vi "LAB4-2.vi"() -> ()   [LabVIEW 2011]
uses:
  <userlib>/KNR LabVIEW Toolkit/General/KNR Open (Direct Mode).vi
  <userlib>/KNR LabVIEW Toolkit/AI Control/AI Library.lvlib
panel:
  out "Voltages":dbl[](array[numeric])
  out "ADC Code":i16[](array[numeric])
  out "Voltage":dbl
  out "Distance (cm)":dbl
  in  "8-15 Single ended":bool=TRUE
  in  "0-7 Single ended":bool=TRUE
  out "error out":errorcluster
  in  "stop":bool
  # "Takes AI0 and converts voltage to distance.\n\n將超音波感測器接上AI0，選擇Sharp型號，\n並轉換為距離。"
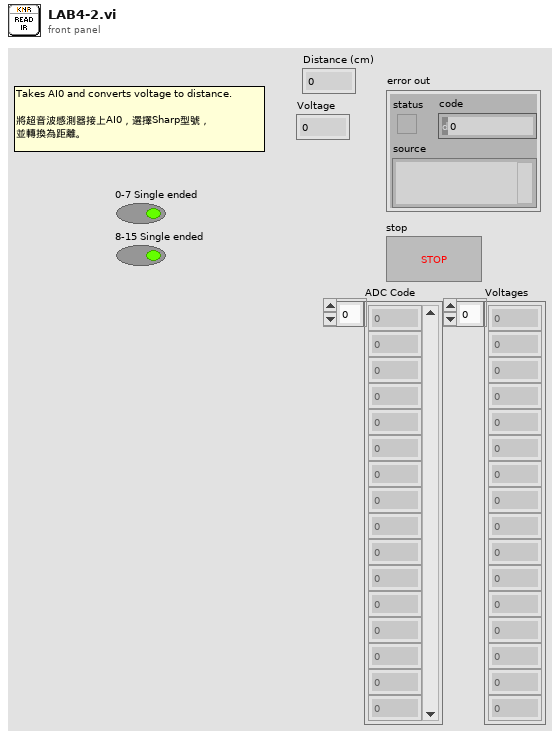
[diagram p1: front panel]
types:
  T1 = typedef "KNR Reference.ctl" = cluster{"FPGA Session":refnum<class "FPGA Interface Base.lvclass">, "Port Types":T2[]}
  T2 = typedef "Port Type (API).ctl" = enum8{"Unassigned", "DIO", "DC Motor", "RC Motor", "Ultrasonic", "Analog Input"}
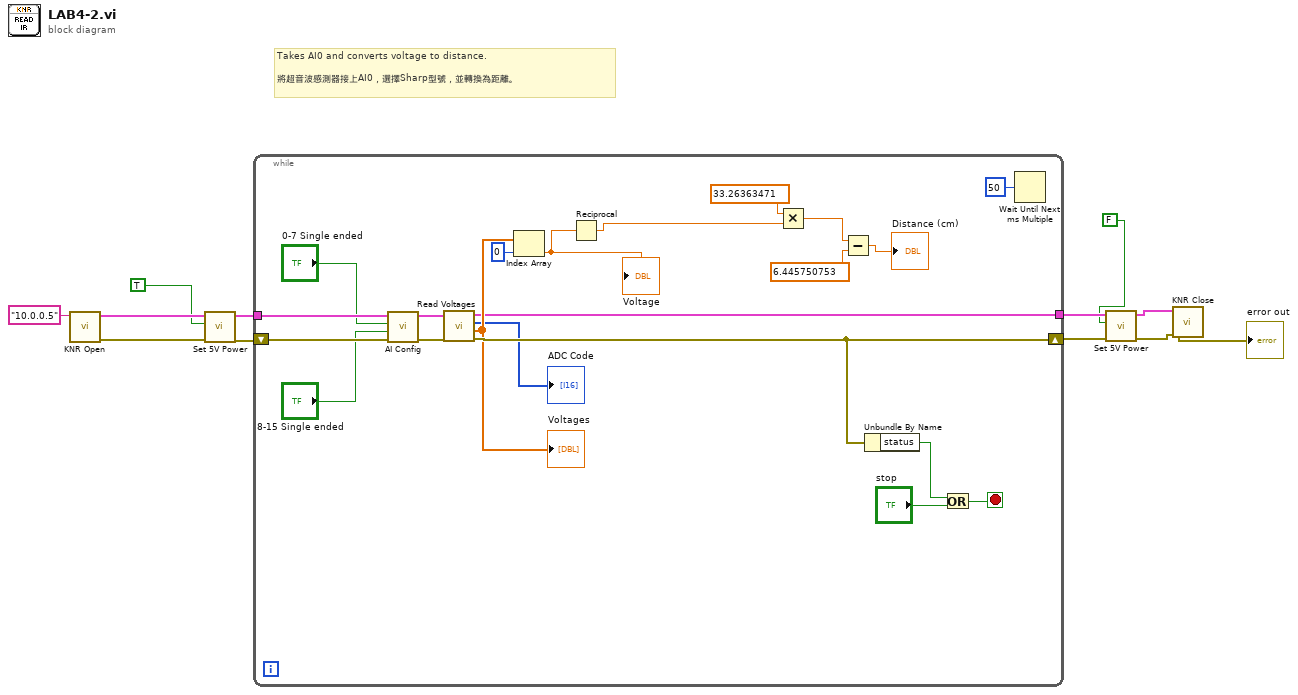
[diagram p0: block diagram]
diagram:
  # "Takes AI0 and converts voltage to distance.\n\n將超音波感測器接上AI0，選擇Sharp型號，並轉換為距離。"
  n1 = call-poly <userlib>:"KNR Open.vi"("IP Address (Default: 10.0.0.5)"="10.0.0.5") -> ("error out"=w11:errorcluster, "KNR Out"=w12:T1)  [unwired: 9 in]
  n2 = call <userlib>:"Set 5V Power.vi"("error in (no error)"=w11, "5V Power"=TRUE, "KNR In"=w12) -> ("error out"=w8:errorcluster, "KNR Out"=w9:T1)  [unwired: 7 in]
  n3 = while {
    tunnel: w9 -> [w29]
    shift-right: [w25] -> w2
    shift-left: w8 -> [w28]
    tunnel: [w14] -> w5
    stop <- w31 stop-if-true
    n4 = call <userlib>:"AI Config.vi"("error in (no error)"=w28, "8-15 Single ended"="8-15 Single ended", "0-7 Single ended"="0-7 Single ended", "KNR In"=w29) -> ("error out"=w26:errorcluster, "KNR Out"=w27:T1)  [unwired: 6 in]
    n5 = call <userlib>:"Read Voltages.vi"("error in (no error)"=w26, "KNR In"=w27) -> ("error out"=w25:errorcluster, "Voltages"=w22:dbl[], "ADC Code"=→"ADC Code":i16[], "KNR Out"=w14:T1)  [unwired: 6 in]
    "Voltages" <- w22
    n6 = Index Array(array=w22, index=0) -> (element=w20:dbl)
    "Voltage" <- w20
    n7 = Reciprocal(x=w20) -> (1/x=w15:dbl)
    n8 = Multiply(x=33.26363471, y=w15) -> (x*y=w17:dbl)
    n9 = Subtract(x=w17, y=6.445750753) -> (x-y=→"Distance (cm)":dbl)
    n10 = Unbundle By Name(w25) -> ("status"=w33:bool)
    n11 = Or(x=w33, y="stop") -> (x .or. y?=w31:bool)
    n12 = Wait Until Next ms Multiple(millisecond multiple=u32 50) -> ()  [unwired: 1 out]
  }
  n13 = call <userlib>:"Set 5V Power.vi"("error in (no error)"=w2, "5V Power"=FALSE, "KNR In"=w5) -> ("error out"=w3:errorcluster, "KNR Out"=w4:T1)  [unwired: 7 in]
  n14 = call <userlib>:"KNR Close.vi"("error in (no error)"=w3, "KNR In"=w4) -> ("error out"=→"error out":errorcluster)  [unwired: 9 in]
